vi "Test Animal Cannot Eat after Eating.vi"(8 "error in (no error)":errorcluster, 11 "Animal Test In":refnum<class "Animal Test.lvclass">) -> (0 "error out":errorcluster, 3 "Animal Test Out":refnum<class "Animal Test.lvclass">)   [LabVIEW 2020, in "Animal Test.lvclass"]
doc: "Test Animal cannot eat after eating."
uses:
  Animal Test.lvclass
  C:/Git/astemes-lunit/source/Framework/Test Case/LUnit Test Case.lvclass
  Animal Test.lvclass/Animal Test.ctl
  Framework/Test Case/LUnit Test Case.lvclass/LUnit Test Case.ctl
  2ca9b3fa-92cf-461f-b55f-c7dec04d1b8c.vi
  Framework/Test Case/Assertions/Fail.vi
  Framework/Test Case/Assertions/Pass.vi
  Framework/Test Case/Private/SubVIs/Compare Variants.vi
  Framework/Test Case/Private/SubVIs/Describe Comparison.vi
  Framework/Test Case/Private/SubVIs/Set Assertion Type.vi
  Framework/Test Case/Private/SubVIs/Add test result.vi
  Framework/Test Case/Private/SubVIs/Variant to string.vi
  Framework/Result Types/Case Result/Public/Record Assertion Result.vi
  Framework/Result Types/Method Result/Public/Aggregate Assertion Results.vi
  Framework/Result Types/Method Result/Private/Merge Status.vi
  Framework/Result Types/Method Result/Private/Concatenate result strings.vi
  <vilib>/Utility/Data Type/Get Type Information.vi
  <vilib>/Utility/LVClass/Get LV Class Name.vi
  Animal Classes/Animal/Animal.lvclass
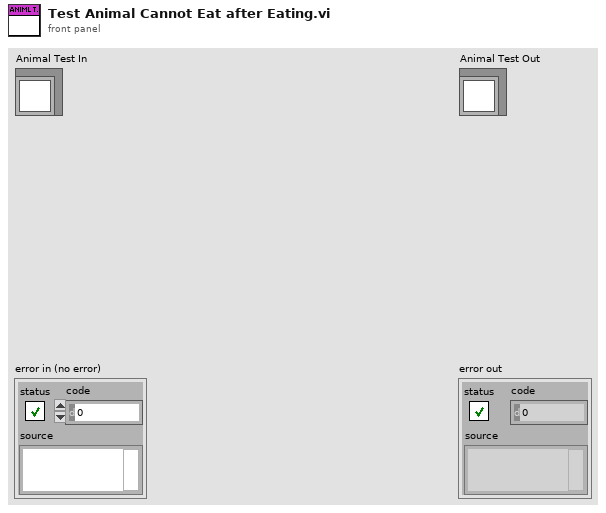
[diagram p1: front panel]
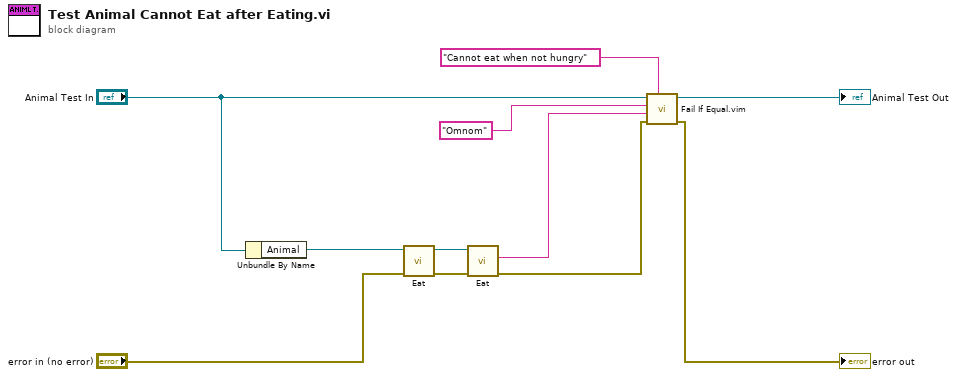
[diagram p0: block diagram]
diagram:
  n1 = Unbundle By Name("Animal Test In") -> ("Animal"=w11:refnum<class "Animal.lvclass">)
  n2 = call-dynamic "Eat.vi"("error in (no error)"="error in (no error)", "Animal In"=w11) -> ("error out"=w9:errorcluster, "Animal Out"=w10:refnum<class "Animal.lvclass">)  [unwired: 7 in, 1 out]
  n3 = call-dynamic "Eat.vi"("error in (no error)"=w9, "Animal In"=w10) -> ("error out"=w2:errorcluster, "Result"=w3:string)  [unwired: 7 in, 1 out]
  n4 = call "Fail If Equal.vim"("Description"="Cannot eat when not hungry", "error in (no error)"=w2, "Actual"=w3, "Expected"="Omnom" ("Result"), "LUnit Test Case In"="Animal Test In") -> ("error out"=→"error out":errorcluster, "LUnit Test Case Out"=→"Animal Test Out":refnum<class "Animal Test.lvclass">)  [unwired: 5 in]
